vi "rsscope_core_global.vi"() -> ()   [LabVIEW 2014] (continued)
Repeated Capabilities:\nNone\n\nRemote-control command(s):\nSEARch:TRIGger:FLXRay:DPOSition"}, {"Level"=4, "Class Only"=FALSE, "Identifier"="RSSCOPE_ATTR_SEARCH_FLEXRAY_DATA_POSITION_MAX", "Descriptive Name"="Search FlexRay Data Position Max", "Data Type"=0, "Command"="SEAR:TRIG:FLXR:DPTO", "Access"=2, "Range Table"="RsScope_rngSearchFlexRayDataPositionMinMax", "Read Callback"="rsscope_FormatSearchNameInt32_ReadCallback.vi", "Write Callback"="rsscope_FormatSearchNameInt32_WriteCallback.vi", "Supported Models"="", "Instrument Options"="", "Flags"=0, "Help"="Defines the last byte of interest, if the position operator RSSCOPE_ATTR_SEARCH_FLEXRAY_DATA_POSITION_CONDITION defines a range.\n\nAvailable Repeated Capabilities:\nNone\n\nRemote-control command(s):\nSEARch:TRIGger:FLXRay:DPTO"}, {"Level"=4, "Class Only"=FALSE, "Identifier"="RSSCOPE_ATTR_SEARCH_FLEXRAY_DATA_CONDITION", "Descriptive Name"="Search FlexRay Data Condition", "Data Type"=0, "Command"="SEAR:TRIG:FLXR:DCON", "Access"=2, "Range Table"="rsscope_rngFlexRayCondition", "Read Callback"="rsscope_FormatSearchNameInt32_ReadCallback.vi", "Write Callback"="rsscope_FormatSearchNameInt32_WriteCallback.vi", "Supported Models"="", "Instrument Options"="", "Flags"=0, "Help"="Sets the operator to set a specific data pattern or a data pattern range.\n\nAvailable Repeated Capabilities:\nNone\n\nRemote-control command(s):\nSEARch:TRIGger:FLXRay:DCONdition"}, {"Level"=4, "Class Only"=FALSE, "Identifier"="RSSCOPE_ATTR_SEARCH_FLEXRAY_DATA_MIN", "Descriptive Name"="Search FlexRay Data Min", "Data Type"=2, "Command"="SEAR:TRIG:FLXR:DMIN", "Access"=1, "Range Table"="", "Read Callback"="", "Write Callback"="rsscope_FormatSearchNameString_WriteCallback.vi", "Supported Models"="", "Instrument Options"="", "Flags"=0, "Help"="Specifies a data pattern, or sets the start value of a data pattern range.\n\nAvailable Repeated Capabilities:\nNone\n\nRemote-control command(s):\nSEARch:TRIGger:FLXRay:DMIN"}, {"Level"=4, "Class Only"=FALSE, "Identifier"="RSSCOPE_ATTR_SEARCH_FLEXRAY_DATA_MAX", "Descriptive Name"="Search FlexRay Data Max", "Data Type"=2, "Command"="SEAR:TRIG:FLXR:DMAX", "Access"=1, "Range Table"="", "Read Callback"="", "Write Callback"="rsscope_FormatSearchNameString_WriteCallback.vi", "Supported Models"="", "Instrument Options"="", "Flags"=0, "Help"="Sets the end value of an data range if RSSCOPE_ATTR_SEARCH_FLEXRAY_DATA_CONDITION is set to In Range or Out Of Range.\n\nAvailable Repeated Capabilities:\nNone\n\nRemote-control command(s):\nSEARch:TRIGger:FLXRay:DMAX"}, {"Level"=4, "Class Only"=FALSE, "Identifier"="RSSCOPE_ATTR_SEARCH_FLEXRAY_IDENTIFIER_MIN", "Descriptive Name"="Search FlexRay Identifier Min", "Data Type"=2, "Command"="SEAR:TRIG:FLXR:IMIN", "Access"=2, "Range Table"="", "Read Callback"="rsscope_FormatSearchNameString_ReadCallback.vi", "Write Callback"="rsscope_FormatSearchNameString_WriteCallback.vi", "Supported Models"="", "Instrument Options"="", "Flags"=0, "Help"="Specifies a identifier pattern, or sets the start value of a identifier pattern range.\n\nAvailable Repeated Capabilities:\nNone\n\nRemote-control command(s):\nSEARch:TRIGger:FLXRay:IMIN"}, {"Level"=4, "Class Only"=FALSE, "Identifier"="RSSCOPE_ATTR_SEARCH_FLEXRAY_IDENTIFIER_MAX", "Descriptive Name"="Search FlexRay Identifier Max", "Data Type"=2, "Command"="SEAR:TRIG:FLXR:IMAX", "Access"=2, "Range Table"="", "Read Callback"="rsscope_FormatSearchNameString_ReadCallback.vi", "Write Callback"="rsscope_FormatSearchNameString_WriteCallback.vi", "Supported Models"="", "Instrument Options"="", "Flags"=0, "Help"="Sets the end value of an identifier range.\n\nAvailable Repeated Capabilities:\nNone\n\nRemote-control command(s):\nSEARch:TRIGger:FLXRay:IMAX"}, {"Level"=4, "Class Only"=FALSE, "Identifier"="RSSCOPE_ATTR_SEARCH_FLEXRAY_SYMBOL", "Descriptive Name"="Search FlexRay Symbol", "Data Type"=0, "Command"="SEAR:TRIG:FLXR:SYMB", "Access"=2, "Range Table"="rsscope_rngFlexRaySymbol", "Read Callback"="rsscope_FormatSearchNameInt32_ReadCallback.vi", "Write Callback"="rsscope_FormatSearchNameInt32_WriteCallback.vi", "Supported Models"="", "Instrument Options"="", "Flags"=0, "Help"="Searches for a symbol or for a wakeup pattern.\n\nAvailable Repeated Capabilities:\nNone\n\nRemote-control command(s):\nSEARch:TRIGger:FLXRay:SYMBol"}, {"Level"=4, "Class Only"=FALSE, "Identifier"="RSSCOPE_ATTR_SEARCH_FLEXRAY_FRAME_START_SEQUENCE_ERROR", "Descriptive Name"="Search FlexRay Frame Start Sequence Error", "Data Type"=3, "Command"="SEAR:TRIG:FLXR:FSS", "Access"=2, "Range Table"="", "Read Callback"="rsscope_FormatSearchNameBoolean_ReadCallback.vi", "Write Callback"="rsscope_FormatSearchNameBoolean_WriteCallback.vi", "Supported Models"="", "Instrument Options"="", "Flags"=0, "Help"="Searches for an error in a Frame Start Sequence(FSS). FSS follows the Transmission Start Sequence (TSS) at the beginning of each frame.\n\nAvailable Repeated Capabilities:\nNone\n\nRemote-control command(s):\nSEARch:TRIGger:FLXRay:FSSerror"}, {"Level"=4, "Class Only"=FALSE, "Identifier"="RSSCOPE_ATTR_SEARCH_FLEXRAY_BYTE_START_SEQUENCE_ERROR", "Descriptive Name"="Search FlexRay Byte Start Sequence Error", "Data Type"=3, "Command"="SEAR:TRIG:FLXR:BSS", "Access"=2, "Range Table"="", "Read Callback"="rsscope_FormatSearchNameBoolean_ReadCallback.vi", "Write Callback"="rsscope_FormatSearchNameBoolean_WriteCallback.vi", "Supported Models"="", "Instrument Options"="", "Flags"=0, "Help"="Searches for error in SyteStart Sequence. The BSS is transmitted before each byte.\n\nAvailable Repeated Capabilities:\nNone\n\nRemote-control command(s):\nSEARch:TRIGger:FLXRay:BSSerror"}, {"Level"=4, "Class Only"=FALSE, "Identifier"="RSSCOPE_ATTR_SEARCH_FLEXRAY_FRAME_END_SEQUENCE_ERROR", "Descriptive Name"="Search FlexRay Frame End Sequence Error", "Data Type"=3, "Command"="SEAR:TRIG:FLXR:FES", "Access"=2, "Range Table"="", "Read Callback"="rsscope_FormatSearchNameBoolean_ReadCallback.vi", "Write Callback"="rsscope_FormatSearchNameBoolean_WriteCallback.vi", "Supported Models"="", "Instrument Options"="", "Flags"=0, "Help"="Searches for error in Frame End Sequence. FES indicates the end of each frame.\n\nAvailable Repeated Capabilities:\nNone\n\nRemote-control command(s):\nSEARch:TRIGger:FLXRay:FESerror"}, {"Level"=4, "Class Only"=FALSE, "Identifier"="RSSCOPE_ATTR_SEARCH_FLEXRAY_HEADER_CRC_ERROR", "Descriptive Name"="Search FlexRay Header CRC Error", "Data Type"=3, "Command"="SEAR:TRIG:FLXR:HCRC", "Access"=2, "Range Table"="", "Read Callback"="rsscope_FormatSearchNameBoolean_ReadCallback.vi", "Write Callback"="rsscope_FormatSearchNameBoolean_WriteCallback.vi", "Supported Models"="", "Instrument Options"="", "Flags"=0, "Help"="Searches for an error in the Cyclic Redundancy Check of the header data (mainly frame ID and payload length).\n\nAvailable Repeated Capabilities:\nNone\n\nRemote-control command(s):\nSEARch:TRIGger:FLXRay:HCRCerror"}, {"Level"=4, "Class Only"=FALSE, "Identifier"="RSSCOPE_ATTR_SEARCH_FLEXRAY_PAYLOAD_CRC_ERROR", "Descriptive Name"="Search FlexRay Payload CRC Error", "Data Type"=3, "Command"="SEAR:TRIG:FLXR:PCRC", "Access"=2, "Range Table"="", "Read Callback"="rsscope_FormatSearchNameBoolean_ReadCallback.vi", "Write Callback"="rsscope_FormatSearchNameBoolean_WriteCallback.vi", "Supported Models"="", "Instrument Options"="", "Flags"=0, "Help"="Searches for error in the Cyclic Redundancy Check of the payload data.\n\nAvailable Repeated Capabilities:\nNone\n\nRemote-control command(s):\nSEARch:TRIGger:FLXRay:PCRCerror"}, {"Level"=3, "Class Only"=TRUE, "Identifier"="", "Descriptive Name"="MIL1553", "Data Type"=0, "Command"="", "Access"=0, "Range Table"="", "Read Callback"="", "Write Callback"="", "Supported Models"="", "Instrument Options"="", "Flags"=0, "Help"="Configures MIL1553 search settings."}, {"Level"=4, "Class Only"=FALSE, "Identifier"="RSSCOPE_ATTR_SEARCH_MIL1553_MODE", "Descriptive Name"="Search MIL1553 Mode", "Data Type"=0, "Command"="SEAR:TRIG:MILS:TYPE", "Access"=2, "Range Table"="rsscope_rngProtocolMIL1553TriggerMode", "Read Callback"="rsscope_FormatSearchNameInt32_ReadCallback.vi", "Write Callback"="rsscope_FormatSearchNameInt32_WriteCallback.vi", "Supported Models"="RTO|RTP", "Instrument Options"="", "Flags"=0, "Help"="Sets the event to be searched for.\n\nAvailable Repeated Capabilities:\nNone\n\nRemote-control command(s):\nSEARch:TRIGger:MILStd:TYPE"}, {"Level"=4, "Class Only"=FALSE, "Identifier"="RSSCOPE_ATTR_SEARCH_MIL1553_SYNC_TYPE", "Descriptive Name"="Search MIL1553 Sync Type", "Data Type"=0, "Command"="SEAR:TRIG:MILS:TPSP", "Access"=2, "Range Table"="rsscope_rngProtocolMIL1553SyncType", "Read Callback"="rsscope_FormatSearchNameInt32_ReadCallback.vi", "Write Callback"="rsscope_FormatSearchNameInt32_WriteCallback.vi", "Supported Models"="RTO|RTP", "Instrument Options"="", "Flags"=0, "Help"="Sets the sync impulse/ word type to be searched for.\n\nAvailable Repeated Capabilities:\nNone\n\nRemote-control command(s):\nSEARch:TRIGger:MILStd:TPSPecifier"}, {"Level"=4, "Class Only"=TRUE, "Identifier"="", "Descriptive Name"="Data", "Data Type"=0, "Command"="", "Access"=0, "Range Table"="", "Read Callback"="", "Write Callback"="", "Supported Models"="", "Instrument Options"="", "Flags"=0, "Help"="Configures MIL1553 search data settings."}, {"Level"=5, "Class Only"=TRUE, "Identifier"="", "Descriptive Name"="Pattern", "Data Type"=0, "Command"="", "Access"=0, "Range Table"="", "Read Callback"="", "Write Callback"="", "Supported Models"="", "Instrument Options"="", "Flags"=0, "Help"="Configures MIL1553 search data pattern settings."}, {"Level"=6, "Class Only"=FALSE, "Identifier"="RSSCOPE_ATTR_SEARCH_MIL1553_DATA_PATTERN_CONDITION", "Descriptive Name"="Search MIL1553 Data Pattern Condition", "Data Type"=0, "Command"="SEAR:TRIG:MILS:DATA:DCON", "Access"=2, "Range Table"="rsscope_rngProtocolMIL1553DataOperator", "Read Callback"="rsscope_FormatSearchNameInt32_ReadCallback.vi", "Write Callback"="rsscope_FormatSearchNameInt32_WriteCallback.vi", "Supported Models"="RTO|RTP", "Instrument Options"="", "Flags"=0, "Help"="Sets the operator to set a specific data pattern.\n\nAvailable Repeated Capabilities:\nNone\n\nRemote-control command(s):\nSEARch:TRIGger:MILStd:DATA:DCONdition"}, {"Level"=6, "Class Only"=FALSE, "Identifier"="RSSCOPE_ATTR_SEARCH_MIL1553_DATA_PATTERN_MIN", "Descriptive Name"="Search MIL1553 Data Pattern Min", "Data Type"=2, "Command"="SEAR:TRIG:MILS:DATA:DMIN", "Access"=1, "Range Table"="", "Read Callback"="", "Write Callback"="rsscope_FormatSearchNameString_WriteCallback.vi", "Supported Models"="RTO|RTP", "Instrument Options"="", "Flags"=0, "Help"="Sets the pattern or the start value of a pattern range for the corresponding data pattern in a data word search.\n\nAvailable Repeated Capabilities:\nNone\n\nRemote-control command(s):\nSEARch:TRIGger:MILStd:DATA:DMIN"}, {"Level"=6, "Class Only"=FALSE, "Identifier"="RSSCOPE_ATTR_SEARCH_MIL1553_DATA_PATTERN_MAX", "Descriptive Name"="Search MIL1553 Data Pattern Max", "Data Type"=2, "Command"="SEAR:TRIG:MILS:DATA:DMAX", "Access"=1, "Range Table"="", "Read Callback"="", "Write Callback"="rsscope_FormatSearchNameString_WriteCallback.vi", "Supported Models"="RTO|RTP", "Instrument Options"="", "Flags"=0, "Help"="Sets the end value of a data pattern range if &apos;Data Pattern Condition&apos; is set to InRange or OutOfRange.\n\nAvailable Repeated Capabilities:\nNone\n\nRemote-control command(s):\nSEARch:TRIGger:MILStd:DATA:DMAX"}, {"Level"=5, "Class Only"=TRUE, "Identifier"="", "Descriptive Name"="Index", "Data Type"=0, "Command"="", "Access"=0, "Range Table"="", "Read Callback"="", "Write Callback"="", "Supported Models"="", "Instrument Options"="", "Flags"=0, "Help"="Configures MIL1553 search data index settings."}, {"Level"=6, "Class Only"=FALSE, "Identifier"="RSSCOPE_ATTR_SEARCH_MIL1553_DATA_INDEX_CONDITION", "Descriptive Name"="Search MIL1553 Data Index Condition", "Data Type"=0, "Command"="SEAR:TRIG:MILS:DATA:ICON", "Access"=2, "Range Table"="rsscope_rngProtocolIndexCondition", "Read Callback"="rsscope_FormatSearchNameInt32_ReadCallback.vi", "Write Callback"="rsscope_FormatSearchNameInt32_WriteCallback.vi", "Supported Models"="RTO|RTP", "Instrument Options"="", "Flags"=0, "Help"="Sets the operator to set a range within a series of the data words that is considered for the search.\n\nAvailable Repeated Capabilities:\nNone\n\nRemote-control command(s):\nSEARch:TRIGger:MILStd:DATA:ICONdition"}, {"Level"=6, "Class Only"=FALSE, "Identifier"="RSSCOPE_ATTR_SEARCH_MIL1553_DATA_INDEX_MIN", "Descriptive Name"="Search MIL1553 Data Index Min", "Data Type"=0, "Command"="SEAR:TRIG:MILS:DATA:IMIN", "Access"=2, "Range Table"="rsscope_rngProtocolMIL1553TriggerDataIndexRange", "Read Callback"="rsscope_FormatSearchNameInt32_ReadCallback.vi", "Write Callback"="rsscope_FormatSearchNameInt32_WriteCallback.vi", "Supported Models"="RTO|RTP", "Instrument Options"="", "Flags"=0, "Help"="Specifies an index or sets the start value of a data word series index range.\n\nAvailable Repeated Capabilities:\nNone\n\nRemote-control command(s):\nSEARch:TRIGger:MILStd:DATA:IMIN"}, {"Level"=6, "Class Only"=FALSE, "Identifier"="RSSCOPE_ATTR_SEARCH_MIL1553_DATA_INDEX_MAX", "Descriptive Name"="Search MIL1553 Data Index Max", "Data Type"=0, "Command"="SEAR:TRIG:MILS:DATA:IMAX", "Access"=2, "Range Table"="rsscope_rngProtocolMIL1553TriggerDataIndexRange", "Read Callback"="rsscope_FormatSearchNameInt32_ReadCallback.vi", "Write Callback"="rsscope_FormatSearchNameInt32_WriteCallback.vi", "Supported Models"="RTO|RTP", "Instrument Options"="", "Flags"=0, "Help"="Sets the end value of a data word series index range if &apos;Data Index Condition&apos; is set to InRange.\n\nAvailable Repeated Capabilities:\nNone\n\nRemote-control command(s):\nSEARch:TRIGger:MILStd:DATA:IMAX"}, {"Level"=5, "Class Only"=TRUE, "Identifier"="", "Descriptive Name"="RTA Pattern", "Data Type"=0, "Command"="", "Access"=0, "Range Table"="", "Read Callback"="", "Write Callback"="", "Supported Models"="", "Instrument Options"="", "Flags"=0, "Help"="Configures MIL1553 search data RTA pattern settings."}, {"Level"=6, "Class Only"=FALSE, "Identifier"="RSSCOPE_ATTR_SEARCH_MIL1553_RTA_DATA_PATTERN_CONDITION", "Descriptive Name"="Search MIL1553 RTA Data Pattern Condition", "Data Type"=0, "Command"="SEAR:TRIG:MILS:DATA:RCON", "Access"=2, "Range Table"="rsscope_rngProtocolMIL1553DataOperator", "Read Callback"="rsscope_FormatSearchNameInt32_ReadCallback.vi", "Write Callback"="rsscope_FormatSearchNameInt32_WriteCallback.vi", "Supported Models"="RTO|RTP", "Instrument Options"="", "Flags"=0, "Help"="Sets the operator to set a specific remote terminal address.\n\nAvailable Repeated Capabilities:\nNone\n\nRemote-control command(s):\nSEARch:TRIGger:MILStd:DATA:RCONdition"}, {"Level"=6, "Class Only"=FALSE, "Identifier"="RSSCOPE_ATTR_SEARCH_MIL1553_RTA_DATA_PATTERN_MIN", "Descriptive Name"="Search MIL1553 RTA Data Pattern Min", "Data Type"=2, "Command"="SEAR:TRIG:MILS:DATA:RMIN", "Access"=1, "Range Table"="", "Read Callback"="", "Write Callback"="rsscope_FormatSearchNameString_WriteCallback.vi", "Supported Models"="RTO|RTP", "Instrument Options"="", "Flags"=0, "Help"="Specifies a remote terminal address or sets the start value of a remote terminal address range.\n\nAvailable Repeated Capabilities:\nNone\n\nRemote-control command(s):\nSEARch:TRIGger:MILStd:DATA:RMIN"}, {"Level"=6, "Class Only"=FALSE, "Identifier"="RSSCOPE_ATTR_SEARCH_MIL1553_RTA_DATA_PATTERN_MAX", "Descriptive Name"="Search MIL1553 RTA Data Pattern Max", "Data Type"=2, "Command"="SEAR:TRIG:MILS:DATA:RMAX", "Access"=1, "Range Table"="", "Read Callback"="", "Write Callback"="rsscope_FormatSearchNameString_WriteCallback.vi", "Supported Models"="RTO|RTP", "Instrument Options"="", "Flags"=0, "Help"="Sets the end value of a data range if &apos;Condition&apos; is set to InRange or OutOfRange.\n\nAvailable Repeated Capabilities:\nNone\n\nRemote-control command(s):\nSEARch:TRIGger:MILStd:DATA:RMAX"}, {"Level"=4, "Class Only"=TRUE, "Identifier"="", "Descriptive Name"="Command Status", "Data Type"=0, "Command"="", "Access"=0, "Range Table"="", "Read Callback"="", "Write Callback"="", "Supported Models"="", "Instrument Options"="", "Flags"=0, "Help"="Configures MIL1553 search command status word settings."}, {"Level"=5, "Class Only"=TRUE, "Identifier"="", "Descriptive Name"="Remote Terminal Address", "Data Type"=0, "Command"="", "Access"=0, "Range Table"="", "Read Callback"="", "Write Callback"="", "Supported Models"="", "Instrument Options"="", "Flags"=0, "Help"="Configures MIL1553 search remote terminal address settings."}, {"Level"=6, "Class Only"=FALSE, "Identifier"="RSSCOPE_ATTR_SEARCH_MIL1553_COMMAND_STATUS_RTA_PATTERN_CONDITION", "Descriptive Name"="Search MIL1553 Command Status RTA Pattern Condition", "Data Type"=0, "Command"="SEAR:TRIG:MILS:CDST:RCON", "Access"=2, "Range Table"="rsscope_rngProtocolMIL1553RTAOperator", "Read Callback"="rsscope_FormatSearchNameInt32_ReadCallback.vi", "Write Callback"="rsscope_FormatSearchNameInt32_WriteCallback.vi", "Supported Models"="RTO|RTP", "Instrument Options"="", "Flags"=0, "Help"="Sets the operator to set a specific remote terminal address.\n\nAvailable Repeated Capabilities:\nNone\n\nRemote-control command(s):\nSEARch:TRIGger:MILStd:CDST:RCONdition"}, {"Level"=6, "Class Only"=FALSE, "Identifier"="RSSCOPE_ATTR_SEARCH_MIL1553_COMMAND_STATUS_RTA_PATTERN_MIN", "Descriptive Name"="Search MIL1553 Command Status RTA Pattern Min", "Data Type"=2, "Command"="SEAR:TRIG:MILS:CDST:RMIN", "Access"=1, "Range Table"="", "Read Callback"="", "Write Callback"="rsscope_FormatSearchNameString_WriteCallback.vi", "Supported Models"="RTO|RTP", "Instrument Options"="", "Flags"=0, "Help"="Specifies a remote terminal address or sets the start value of a remote terminal address range.\n\nAvailable Repeated Capabilities:\nNone\n\nRemote-control command(s):\nSEARch:TRIGger:MILStd:CDST:RMIN"}, {"Level"=6, "Class Only"=FALSE, "Identifier"="RSSCOPE_ATTR_SEARCH_MIL1553_COMMAND_STATUS_RTA_PATTERN_MAX", "Descriptive Name"="Search MIL1553 Command Status RTA Pattern Max", "Data Type"=2, "Command"="SEAR:TRIG:MILS:CDST:RMAX", "Access"=1, "Range Table"="", "Read Callback"="", "Write Callback"="rsscope_FormatSearchNameString_WriteCallback.vi", "Supported Models"="RTO|RTP", "Instrument Options"="", "Flags"=0, "Help"="Sets the end value of a data range if &apos;RTA Condition&apos; is set to InRange or OutOfRange.\n\nAvailable Repeated Capabilities:\nNone\n\nRemote-control command(s):\nSEARch:TRIGger:MILStd:CDST:RMAX"}, {"Level"=5, "Class Only"=TRUE, "Identifier"="", "Descriptive Name"="Info", "Data Type"=0, "Command"="", "Access"=0, "Range Table"="", "Read Callback"="", "Write Callback"="", "Supported Models"="", "Instrument Options"="", "Flags"=0, "Help"="Configures MIL1553 search 11-Bit Information settings."}, {"Level"=6, "Class Only"=FALSE, "Identifier"="RSSCOPE_ATTR_SEARCH_MIL1553_INFO_PATTERN_CONDITION", "Descriptive Name"="Search MIL1553 Info Pattern Condition", "Data Type"=0, "Command"="SEAR:TRIG:MILS:CDST:ICON", "Access"=2, "Range Table"="rsscope_rngProtocolMIL1553InfoOperator", "Read Callback"="rsscope_FormatSearchNameInt32_ReadCallback.vi", "Write Callback"="rsscope_FormatSearchNameInt32_WriteCallback.vi", "Supported Models"="RTO|RTP", "Instrument Options"="", "Flags"=0, "Help"="Sets the operator to set a specific info for the 9th to 19th bit of a command or status word.\n\nAvailable Repeated Capabilities:\nNone\n\nRemote-control command(s):\nSEARch:TRIGger:MILStd:CDST:ICONdition"}, {"Level"=6, "Class Only"=FALSE, "Identifier"="RSSCOPE_ATTR_SEARCH_MIL1553_INFO_PATTERN_MIN", "Descriptive Name"="Search MIL1553 Info Pattern Min", "Data Type"=2, "Command"="SEAR:TRIG:MILS:CDST:IMIN", "Access"=1, "Range Table"="", "Read Callback"="", "Write Callback"="rsscope_FormatSearchNameString_WriteCallback.vi", "Supported Models"="RTO|RTP", "Instrument Options"="", "Flags"=0, "Help"="Sets the pattern or the start value of a pattern range for the corresponding search.\n\nAvailable Repeated Capabilities:\nNone\n\nRemote-control command(s):\nSEARch:TRIGger:MILStd:CDST:IMIN"}, {"Level"=6, "Class Only"=FALSE, "Identifier"="RSSCOPE_ATTR_SEARCH_MIL1553_INFO_PATTERN_MAX", "Descriptive Name"="Search MIL1553 Info Pattern Max", "Data Type"=2, "Command"="SEAR:TRIG:MILS:CDST:IMAX", "Access"=1, "Range Table"="", "Read Callback"="rsscope_FormatSearchNameString_ReadCallback.vi", "Write Callback"="rsscope_FormatSearchNameString_WriteCallback.vi", "Supported Models"="RTO|RTP", "Instrument Options"="", "Flags"=0, "Help"="Sets the end value of the info range if &apos;Info Condition&apos; is set to InRange or OutOfRange.\n\nAvailable Repeated Capabilities:\nNone\n\nRemote-control command(s):\nSEARch:TRIGger:MILStd:CDST:IMAX"}, {"Level"=4, "Class Only"=TRUE, "Identifier"="", "Descriptive Name"="Command", "Data Type"=0, "Command"="", "Access"=0, "Range Table"="", "Read Callback"="", "Write Callback"="", "Supported Models"="", "Instrument Options"="", "Flags"=0, "Help"="Configures MIL1553 search command word settings."}, {"Level"=5, "Class Only"=FALSE, "Identifier"="RSSCOPE_ATTR_SEARCH_MIL1553_COMMAND_TRANSMIT_RECEIVE", "Descriptive Name"="Search MIL1553 Command Transmit Receive", "Data Type"=0, "Command"="SEAR:TRIG:MILS:CMD:TR", "Access"=2, "Range Table"="rsscope_rngProtocolMIL1553TriggerCommandTransmitReceive", "Read Callback"="rsscope_FormatSearchNameInt32_ReadCallback.vi", "Write Callback"="rsscope_FormatSearchNameInt32_WriteCallback.vi", "Supported Models"="RTO|RTP", "Instrument Options"="", "Flags"=0, "Help"="Searches for a transmission mode.\n\nAvailable Repeated Capabilities:\nNone\n\nRemote-control command(s):\nSEARch:TRIGger:MILStd:CMD:TR"}, {"Level"=5, "Class Only"=TRUE, "Identifier"="", "Descriptive Name"="Subaddress", "Data Type"=0, "Command"="", "Access"=0, "Range Table"="", "Read Callback"="", "Write Callback"="", "Supported Models"="", "Instrument Options"="", "Flags"=0, "Help"="Configures MIL1553 search subaddress settings."}, {"Level"=6, "Class Only"=FALSE, "Identifier"="RSSCOPE_ATTR_SEARCH_MIL1553_COMMAND_SUBADDRESS_PATTERN_CONDITION", "Descriptive Name"="Search MIL1553 Command Subaddress Pattern Condition", "Data Type"=0, "Command"="SEAR:TRIG:MILS:CMD:SCON", "Access"=2, "Range Table"="rsscope_rngProtocolMIL1553SubaddressOperator", "Read Callback"="rsscope_FormatSearchNameInt32_ReadCallback.vi", "Write Callback"="rsscope_FormatSearchNameInt32_WriteCallback.vi", "Supported Models"="RTO|RTP", "Instrument Options"="", "Flags"=0, "Help"="Sets the operator to set a specific subaddress/mode pattern.\n\nAvailable Repeated Capabilities:\nNone\n\nRemote-control command(s):\nSEARch:TRIGger:MILStd:CMD:SCONdition"}, {"Level"=6, "Class Only"=FALSE, "Identifier"="RSSCOPE_ATTR_SEARCH_MIL1553_COMMAND_SUBADDRESS_PATTERN_MIN", "Descriptive Name"="Search MIL1553 Command Subaddress Pattern Min", "Data Type"=2, "Command"="SEAR:TRIG:MILS:CMD:SMIN", "Access"=1, "Range Table"="", "Read Callback"="", "Write Callback"="rsscope_FormatSearchNameString_WriteCallback.vi", "Supported Models"="RTO|RTP", "Instrument Options"="", "Flags"=0, "Help"="Specifies a subaddress or sets the start value of a subaddress range.\n\nAvailable Repeated Capabilities:\nNone\n\nRemote-control command(s):\nSEARch:TRIGger:MILStd:CMD:SMIN"}, {"Level"=6, "Class Only"=FALSE, "Identifier"="RSSCOPE_ATTR_SEARCH_MIL1553_COMMAND_SUBADDRESS_PATTERN_MAX", "Descriptive Name"="Search MIL1553 Command Subaddress Pattern Max", "Data Type"=2, "Command"="SEAR:TRIG:MILS:CMD:SMAX", "Access"=1, "Range Table"="", "Read Callback"="", "Write Callback"="rsscope_FormatSearchNameString_WriteCallback.vi", "Supported Models"="RTO|RTP", "Instrument Options"="", "Flags"=0, "Help"="Sets the end value of the info subaddress if &apos;Subaddress Condition&apos; is set to InRange or OutOfRange.\n\nAvailable Repeated Capabilities:\nNone\n\nRemote-control command(s):\nSEARch:TRIGger:MILStd:CMD:SMAX"}, {"Level"=5, "Class Only"=TRUE, "Identifier"="", "Descriptive Name"="RTA Pattern", "Data Type"=0, "Command"="", "Access"=0, "Range Table"="", "Read Callback"="", "Write Callback"="", "Supported Models"="", "Instrument Options"="", "Flags"=0, "Help"="Configures MIL1553 search RTA Pattern settings."}, {"Level"=6, "Class Only"=FALSE, "Identifier"="RSSCOPE_ATTR_SEARCH_MIL1553_COMMAND_RTA_PATTERN_CONDITION", "Descriptive Name"="Search MIL1553 Command RTA Pattern Condition", "Data Type"=0, "Command"="SEAR:TRIG:MILS:CMD:RCON", "Access"=2, "Range Table"="rsscope_rngProtocolMIL1553SubaddressOperator", "Read Callback"="rsscope_FormatSearchNameInt32_ReadCallback.vi", "Write Callback"="rsscope_FormatSearchNameInt32_WriteCallback.vi", "Supported Models"="RTO|RTP", "Instrument Options"="", "Flags"=0, "Help"="Sets the operator to define a remote terminal address.\n\nAvailable Repeated Capabilities:\nNone\n\nRemote-control command(s):\nSEARch:TRIGger:MILStd:CMD:RCONdition"}, {"Level"=6, "Class Only"=FALSE, "Identifier"="RSSCOPE_ATTR_SEARCH_MIL1553_COMMAND_RTA_PATTERN_MIN", "Descriptive Name"="Search MIL1553 Command RTA Pattern Min", "Data Type"=2, "Command"="SEAR:TRIG:MILS:CMD:RMIN", "Access"=1, "Range Table"="", "Read Callback"="", "Write Callback"="rsscope_FormatSearchNameString_WriteCallback.vi", "Supported Models"="RTO|RTP", "Instrument Options"="", "Flags"=0, "Help"="Specify a remote terminal address or set the start value of a remote terminal address range.\n\nAvailable Repeated Capabilities:\nNone\n\nRemote-control command(s):\nSEARch:TRIGger:MILStd:CMD:RMIN"}, {"Level"=6, "Class Only"=FALSE, "Identifier"="RSSCOPE_ATTR_SEARCH_MIL1553_COMMAND_RTA_PATTERN_MAX", "Descriptive Name"="Search MIL1553 Command RTA Pattern Max", "Data Type"=2, "Command"="SEAR:TRIG:MILS:CMD:RMAX", "Access"=1, "Range Table"="", "Read Callback"="", "Write Callback"="rsscope_FormatSearchNameString_WriteCallback.vi", "Supported Models"="RTO|RTP", "Instrument Options"="", "Flags"=0, "Help"="Set the end value of a data range  if &apos;Subaddress Condition&apos; is set to InRange or OutOfRange.\n\nAvailable Repeated Capabilities:\nNone\n\nRemote-control command(s):\nSEARch:TRIGger:MILStd:CMD:RMAX"}, {"Level"=5, "Class Only"=TRUE, "Identifier"="", "Descriptive Name"="Word Count", "Data Type"=0, "Command"="", "Access"=0, "Range Table"="", "Read Callback"="", "Write Callback"="", "Supported Models"="", "Instrument Options"="", "Flags"=0, "Help"="Configures MIL1553 search word count/ mode code settings."}, {"Level"=6, "Class Only"=FALSE, "Identifier"="RSSCOPE_ATTR_SEARCH_MIL1553_COMMAND_WORD_COUNT_PATTERN_CONDITION", "Descriptive Name"="Search MIL1553 Command Word Count Pattern Condition", "Data Type"=0, "Command"="SEAR:TRIG:MILS:CMD:CCON", "Access"=2, "Range Table"="rsscope_rngProtocolMIL1553WordCountOperator", "Read Callback"="rsscope_FormatSearchNameInt32_ReadCallback.vi", "Write Callback"="rsscope_FormatSearchNameInt32_WriteCallback.vi", "Supported Models"="RTO|RTP", "Instrument Options"="", "Flags"=0, "Help"="Sets the operator to set a specific data word count or mode code pattern.\n\nAvailable Repeated Capabilities:\nNone\n\nRemote-control command(s):\nSEARch:TRIGger:MILStd:CMD:CCONdition"}, {"Level"=6, "Class Only"=FALSE, "Identifier"="RSSCOPE_ATTR_SEARCH_MIL1553_COMMAND_WORD_COUNT_PATTERN_MIN", "Descriptive Name"="Search MIL1553 Command Word Count Pattern Min", "Data Type"=2, "Command"="SEAR:TRIG:MILS:CMD:CMIN", "Access"=1, "Range Table"="", "Read Callback"="", "Write Callback"="rsscope_FormatSearchNameString_WriteCallback.vi", "Supported Models"="RTO|RTP", "Instrument Options"="", "Flags"=0, "Help"="Specifies a data word count/mode code pattern or sets the start value of a pattern range.\n\nAvailable Repeated Capabilities:\nNone\n\nRemote-control command(s):\nSEARch:TRIGger:MILStd:CMD:CMIN"}, {"Level"=6, "Class Only"=FALSE, "Identifier"="RSSCOPE_ATTR_SEARCH_MIL1553_COMMAND_WORD_COUNT_PATTERN_MAX", "Descriptive Name"="Search MIL1553 Command Word Count Pattern Max", "Data Type"=2, "Command"="SEAR:TRIG:MILS:CMD:CMAX", "Access"=1, "Range Table"="", "Read Callback"="", "Write Callback"="rsscope_FormatSearchNameString_WriteCallback.vi", "Supported Models"="RTO|RTP", "Instrument Options"="", "Flags"=0, "Help"="Sets the end value of a data word count/mode code pattern if &apos;Word Count Condition&apos; is set to InRange or OutOfRange.\n\nAvailable Repeated Capabilities:\nNone\n\nRemote-control command(s):\nSEARch:TRIGger:MILStd:CMD:CMAX"}, {"Level"=4, "Class Only"=TRUE, "Identifier"="", "Descriptive Name"="Status Flags", "Data Type"=0, "Command"="", "Access"=0, "Range Table"="", "Read Callback"="", "Write Callback"="", "Supported Models"="", "Instrument Options"="", "Flags"=0, "Help"="Specifies the values of the status flags. You can use the following characters: 1; 0; or X (don&apos;t care)."}, {"Level"=5, "Class Only"=FALSE, "Identifier"="RSSCOPE_ATTR_SEARCH_MIL1553_STATUS_FLAG_MESSAGE_ERROR", "Descriptive Name"="Search MIL1553 Status Flag Message Error", "Data Type"=0, "Command"="SEAR:TRIG:MILS:STAT:MERR", "Access"=2, "Range Table"="rsscope_rngProtocolMIL1553TriggerStatusFlags", "Read Callback"="rsscope_FormatSearchNameInt32_ReadCallback.vi", "Write Callback"="rsscope_FormatSearchNameInt32_WriteCallback.vi", "Supported Models"="RTO|RTP", "Instrument Options"="", "Flags"=0, "Help"="Searches for the state of the message error bit of the status word if &apos;Trigger Mode&apos; is set to StatusWord.\n\nAvailable Repeated Capabilities:\nNone\n\nRemote-control command(s):\nSEARch:TRIGger:MILStd:STATus:MERRor"}, {"Level"=5, "Class Only"=FALSE, "Identifier"="RSSCOPE_ATTR_SEARCH_MIL1553_STATUS_FLAG_BUSY", "Descriptive Name"="Search MIL1553 Status Flag Busy", "Data Type"=0, "Command"="SEAR:TRIG:MILS:STAT:BUSY", "Access"=2, "Range Table"="rsscope_rngProtocolMIL1553TriggerStatusFlags", "Read Callback"="rsscope_FormatSearchNameInt32_ReadCallback.vi", "Write Callback"="rsscope_FormatSearchNameInt32_WriteCallback.vi", "Supported Models"="RTO|RTP", "Instrument Options"="", "Flags"=0, "Help"="Searches for  the state of the busy bit of the status word if &apos;Trigger Mode&apos; is set to StatusWord.\n\nAvailable Repeated Capabilities:\nNone\n\nRemote-control command(s):\nSEARch:TRIGger:MILStd:STATus:BUSY"}, {"Level"=5, "Class Only"=FALSE, "Identifier"="RSSCOPE_ATTR_SEARCH_MIL1553_STATUS_FLAG_INSTRUMENTATION", "Descriptive Name"="Search MIL1553 Status Flag Instrumentation", "Data Type"=0, "Command"="SEAR:TRIG:MILS:STAT:INST", "Access"=2, "Range Table"="rsscope_rngProtocolMIL1553TriggerStatusFlags", "Read Callback"="rsscope_FormatSearchNameInt32_ReadCallback.vi", "Write Callback"="rsscope_FormatSearchNameInt32_WriteCallback.vi", "Supported Models"="RTO|RTP", "Instrument Options"="", "Flags"=0, "Help"="Searches for  the state of the instrumentation bit of the status word if &apos;Trigger Mode&apos; is set to StatusWord.\n\nAvailable Repeated Capabilities:\nNone\n\nRemote-control command(s):\nSEARch:TRIGger:MILStd:STATus:INSTrument"}, {"Level"=5, "Class Only"=FALSE, "Identifier"="RSSCOPE_ATTR_SEARCH_MIL1553_STATUS_FLAG_SUBSYSTEM", "Descriptive Name"="Search MIL1553 Status Flag Subsystem", "Data Type"=0, "Command"="SEAR:TRIG:MILS:STAT:SUBS", "Access"=2, "Range Table"="rsscope_rngProtocolMIL1553TriggerStatusFlags", "Read Callback"="rsscope_FormatSearchNameInt32_ReadCallback.vi", "Write Callback"="rsscope_FormatSearchNameInt32_WriteCallback.vi", "Supported Models"="RTO|RTP", "Instrument Options"="", "Flags"=0, "Help"="Searches for  the state of the subsystem flag bit of the status word if &apos;Trigger Mode&apos; is set to StatusWord.\n\nAvailable Repeated Capabilities:\nNone\n\nRemote-control command(s):\nSEARch:TRIGger:MILStd:STATus:SUBSystem"}, {"Level"=5, "Class Only"=FALSE, "Identifier"="RSSCOPE_ATTR_SEARCH_MIL1553_STATUS_FLAG_SERVICE_REQUEST", "Descriptive Name"="Search MIL1553 Status Flag Service Request", "Data Type"=0, "Command"="SEAR:TRIG:MILS:STAT:SREQ", "Access"=2, "Range Table"="rsscope_rngProtocolMIL1553TriggerStatusFlags", "Read Callback"="rsscope_FormatSearchNameInt32_ReadCallback.vi", "Write Callback"="rsscope_FormatSearchNameInt32_WriteCallback.vi", "Supported Models"="RTO|RTP", "Instrument Options"="", "Flags"=0, "Help"="Searches for  the state of the service request bit of the status word if &apos;Trigger Mode&apos; is set to StatusWord.\n\nAvailable Repeated Capabilities:\nNone\n\nRemote-control command(s):\nSEARch:TRIGger:MILStd:STATus:SREQuest"}, {"Level"=5, "Class Only"=FALSE, "Identifier"="RSSCOPE_ATTR_SEARCH_MIL1553_STATUS_FLAG_DYNAMIC_BUS_CONTROL", "Descriptive Name"="Search MIL1553 Status Flag Dynamic Bus Control", "Data Type"=0, "Command"="SEAR:TRIG:MILS:STAT:DBC", "Access"=2, "Range Table"="rsscope_rngProtocolMIL1553TriggerStatusFlags", "Read Callback"="rsscope_FormatSearchNameInt32_ReadCallback.vi", "Write Callback"="rsscope_FormatSearchNameInt32_WriteCallback.vi", "Supported Models"="RTO|RTP", "Instrument Options"="", "Flags"=0, "Help"="Searches for  the state of the dynamic bus control accept bit of the status word if &apos;Trigger Mode&apos; is set to StatusWord.\n\nAvailable Repeated Capabilities:\nNone\n\nRemote-control command(s):\nSEARch:TRIGger:MILStd:STATus:DBCaccept"}, {"Level"=5, "Class Only"=FALSE, "Identifier"="RSSCOPE_ATTR_SEARCH_MIL1553_STATUS_FLAG_BROADCAST_COMMAND", "Descriptive Name"="Search MIL1553 Status Flag Broadcast Command", "Data Type"=0, "Command"="SEAR:TRIG:MILS:STAT:BCR", "Access"=2, "Range Table"="rsscope_rngProtocolMIL1553TriggerStatusFlags", "Read Callback"="rsscope_FormatSearchNameInt32_ReadCallback.vi", "Write Callback"="rsscope_FormatSearchNameInt32_WriteCallback.vi", "Supported Models"="RTO|RTP", "Instrument Options"="", "Flags"=0, "Help"="Searches for  the state of the broadcast command received bit of the status word if &apos;Trigger Mode&apos; is set to StatusWord.\n\nAvailable Repeated Capabilities:\nNone\n\nRemote-control command(s):\nSEARch:TRIGger:MILStd:STATus:BCReceived"}, {"Level"=5, "Class Only"=FALSE, "Identifier"="RSSCOPE_ATTR_SEARCH_MIL1553_STATUS_FLAG_TERMINAL", "Descriptive Name"="Search MIL1553 Status Flag Terminal", "Data Type"=0, "Command"="SEAR:TRIG:MILS:STAT:TERM", "Access"=2, "Range Table"="rsscope_rngProtocolMIL1553TriggerStatusFlags", "Read Callback"="rsscope_FormatSearchNameInt32_ReadCallback.vi", "Write Callback"="rsscope_FormatSearchNameInt32_WriteCallback.vi", "Supported Models"="RTO|RTP", "Instrument Options"="", "Flags"=0, "Help"="Searches for  the state of the terminal flag bit of the status word if &apos;Trigger Mode&apos; is set to StatusWord.\n\nAvailable Repeated Capabilities:\nNone\n\nRemote-control command(s):\nSEARch:TRIGger:MILStd:STATus:TERMinal"}, {"Level"=4, "Class Only"=TRUE, "Identifier"="", "Descriptive Name"="Error Condition", "Data Type"=0, "Command"="", "Access"=0, "Range Table"="", "Read Callback"="", "Write Callback"="", "Supported Models"="", "Instrument Options"="", "Flags"=0, "Help"="Specifies the error conditions to be searched for."}, {"Level"=5, "Class Only"=FALSE, "Identifier"="RSSCOPE_ATTR_SEARCH_MIL1553_ERROR_SYNCHRONIZATION_ERROR", "Descriptive Name"="Search MIL1553 Error Synchronization Error", "Data Type"=3, "Command"="SEAR:TRIG:MILS:ERR:SYNC", "Access"=2, "Range Table"="", "Read Callback"="rsscope_FormatSearchNameBoolean_ReadCallback.vi", "Write Callback"="rsscope_FormatSearchNameBoolean_WriteCallback.vi", "Supported Models"="RTO|RTP", "Instrument Options"="", "Flags"=0, "Help"="Searches for an error of the synchronization.\n\nAvailable Repeated Capabilities:\nNone\n\nRemote-control command(s):\nSEARch:TRIGger:MILStd:ERRor:SYNC"}, {"Level"=5, "Class Only"=FALSE, "Identifier"="RSSCOPE_ATTR_SEARCH_MIL1553_ERROR_PARITY_ERROR", "Descriptive Name"="Search MIL1553 Error Parity Error", "Data Type"=3, "Command"="SEAR:TRIG:MILS:ERR:PAR", "Access"=2, "Range Table"="", "Read Callback"="rsscope_FormatSearchNameBoolean_ReadCallback.vi", "Write Callback"="rsscope_FormatSearchNameBoolean_WriteCallback.vi", "Supported Models"="RTO|RTP", "Instrument Options"="", "Flags"=0, "Help"="Checks the parity of every word and searches if the parity is even.\n\nAvailable Repeated Capabilities:\nNone\n\nRemote-control command(s):\nSEARch:TRIGger:MILStd:ERRor:PARity"}, {"Level"=5, "Class Only"=FALSE, "Identifier"="RSSCOPE_ATTR_SEARCH_MIL1553_ERROR_MANCHESTER_CODING_ERROR", "Descriptive Name"="Search MIL1553 Error Manchester Coding Error", "Data Type"=3, "Command"="SEAR:TRIG:MILS:ERR:MANC", "Access"=2, "Range Table"="", "Read Callback"="rsscope_FormatSearchNameBoolean_ReadCallback.vi", "Write Callback"="rsscope_FormatSearchNameBoolean_WriteCallback.vi", "Supported Models"="RTO|RTP", "Instrument Options"="", "Flags"=0, "Help"="Searches if there is an error in the Manchester coding of the signal.\n\nAvailable Repeated Capabilities:\nNone\n\nRemote-control command(s):\nSEARch:TRIGger:MILStd:ERRor:MANChester"}, {"Level"=5, "Class Only"=FALSE, "Identifier"="RSSCOPE_ATTR_SEARCH_MIL1553_ERROR_TIMING_ERROR", "Descriptive Name"="Search MIL1553 Error Timing Error", "Data Type"=3, "Command"="SEAR:TRIG:MILS:ERR:TIM", "Access"=2, "Range Table"="", "Read Callback"="rsscope_FormatSearchNameBoolean_ReadCallback.vi", "Write Callback"="rsscope_FormatSearchNameBoolean_WriteCallback.vi", "Supported Models"="RTO|RTP", "Instrument Options"="", "Flags"=0, "Help"="Checks if the minimum gap is out of range.\n\nAvailable Repeated Capabilities:\nNone\n\nRemote-control command(s):\nSEARch:TRIGger:MILStd:ERRor:TIMing"}, {"Level"=4, "Class Only"=TRUE, "Identifier"="", "Descriptive Name"="Results", "Data Type"=0, "Command"="", "Access"=0, "Range Table"="", "Read Callback"="", "Write Callback"="", "Supported Models"="", "Instrument Options"="", "Flags"=0, "Help"="Returns the search result of the specified word."}, {"Level"=5, "Class Only"=FALSE, "Identifier"="RSSCOPE_ATTR_SEARCH_MIL1553_WORDS_COUNT", "Descriptive Name"="Search MIL1553 Words Count", "Data Type"=0, "Command"="SEAR:RES:MILS:WCO?", "Access"=0, "Range Table"="", "Read Callback"="rsscope_FormatSearchNameInt32_ReadCallback.vi", "Write Callback"="", "Supported Models"="RTO|RTP", "Instrument Options"="", "Flags"=0, "Help"="Returns the number of decoded words.\n\nAvailable Repeated Capabilities:\nNone\n\nRemote-control command(s):\nSEARch:RESult:MILStd:WCOunt?"}, {"Level"=3, "Class Only"=TRUE, "Identifier"="", "Descriptive Name"="ARINC 429", "Data Type"=0, "Command"="", "Access"=0, "Range Table"="", "Read Callback"="", "Write Callback"="", "Supported Models"="", "Instrument Options"="", "Flags"=0, "Help"="Configures ARINC 429 trigger settings."}, {"Level"=4, "Class Only"=FALSE, "Identifier"="RSSCOPE_ATTR_SEARCH_ARINC429_MODE", "Descriptive Name"="Search ARINC429 Mode", "Data Type"=0, "Command"="SEAR:TRIG:ARIN:TYPE", "Access"=2, "Range Table"="rsscope_rngProtocolARINC429TriggerMode", "Read Callback"="rsscope_FormatSearchNameInt32_ReadCallback.vi", "Write Callback"="rsscope_FormatSearchNameInt32_WriteCallback.vi", "Supported Models"="RTO|RTP", "Instrument Options"="", "Flags"=0, "Help"="Sets the search type for ARINC 429 analysis.\n\nAvailable Repeated Capabilities:\nNone\n\nRemote-control command(s):\nSEARch:TRIGger:ARINc:TYPE"}, {"Level"=4, "Class Only"=TRUE, "Identifier"="", "Descriptive Name"="Label Data", "Data Type"=0, "Command"="", "Access"=0, "Range Table"="", "Read Callback"="", "Write Callback"="", "Supported Models"="", "Instrument Options"="", "Flags"=0, "Help"="Configures ARINC 429 search label+data settings."}, {"Level"=5, "Class Only"=FALSE, "Identifier"="RSSCOPE_ATTR_SEARCH_ARINC429_LABEL_DATA_SDI", "Descriptive Name"="Search ARINC429 Label Data SDI", "Data Type"=0, "Command"="SEAR:TRIG:ARIN:SDI", "Access"=1, "Range Table"="", "Read Callback"="", "Write Callback"="rsscope_FormatSearchNameInt32_WriteCallback.vi", "Supported Models"="RTO|RTP", "Instrument Options"="", "Flags"=0, "Help"="Sets the source/destination identifier (SDI) bits.\n\nAvailable Repeated Capabilities:\nNone\n\nRemote-control command(s):\nSEARch:TRIGger:ARINc:SDI"}, {"Level"=5, "Class Only"=FALSE, "Identifier"="RSSCOPE_ATTR_SEARCH_ARINC429_LABEL_DATA_SSM", 
